vi "VerifyPath.vi"(1 "Expected Path":path, 2 "Path To Verify":path) -> (0 "Are Paths Equal?":bool)   [LabVIEW 2012]
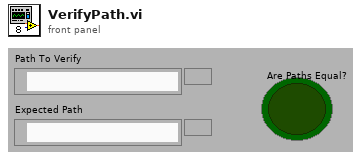
[diagram p1: front panel]
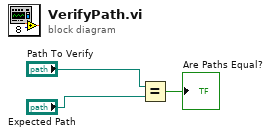
[diagram p0: block diagram]
diagram:
  n1 = Equal?(x="Path To Verify", y="Expected Path") -> (x = y?=→"Are Paths Equal?":bool)
